vi "write_buffer_to_file.vi"(8 "error in (no error)":errorcluster, 10 "data_logger.lvclass":refnum<class "data_logger.lvclass">, 11 "hydraharp in":refnum<class "hydraharp.lvclass">) -> (0 "error out":errorcluster, 1 "stream_done":bool, 2 "data_logger.lvclass 2":refnum<class "data_logger.lvclass">, 3 "hydraharp out":refnum<class "hydraharp.lvclass">)   [LabVIEW 2015, in "hydraharp.lvclass"]
uses:
  hydraharp.lvclass
  Data Logger Class/data_logger.lvclass
  hydraharp.lvclass/hydraharp.ctl
  lvoop_dll-master/picoquant_Tmodes.ctl
  lvoop_dll-master/picoquant_devices.ctl
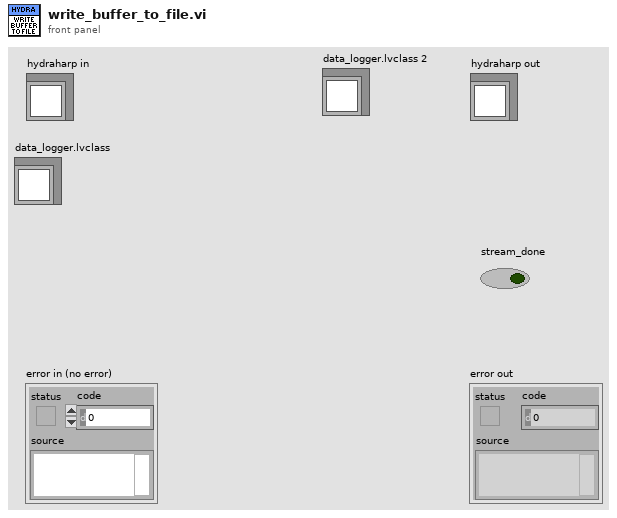
[diagram p1: front panel]
types:
  T1 = typedef "picoquant_devices.ctl" = enum16{"hydraharp", "picoharp"}
  T2 = typedef "hpanel_acq_modes.ctl" = u16
  T3 = typedef "picoquant_Tmodes.ctl" = u16
  T4 = typedef "hydraharp_fifo_queue_data.ctl" = cluster{"fifo_buffer":u32[], "fifo_action":T5}
  T5 = typedef "hydraharp_fifo_actions.ctl" = enum16{"stop", "new_data"}
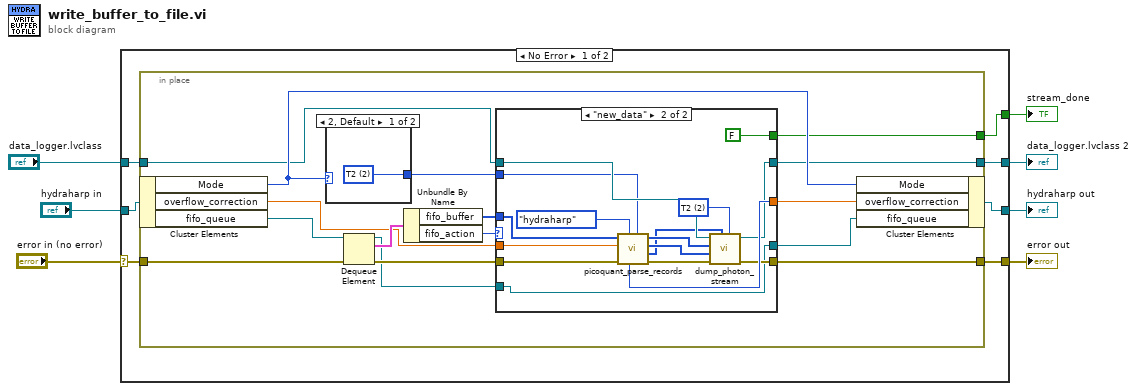
[diagram p0: block diagram]
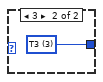
[diagram p2: hidden frame]
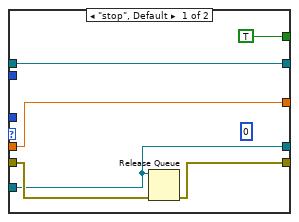
[diagram p3: hidden frame]
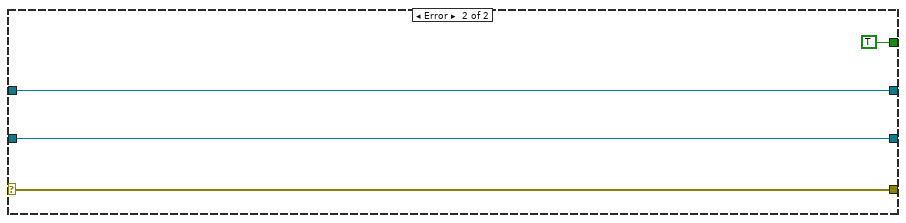
[diagram p4: hidden frame]
diagram:
  n1 = case shown="No Error" "error in (no error)" {
    selector: "error in (no error)" -> [w13 w55]
    tunnel: "data_logger.lvclass" -> [w9 w58]
    tunnel: "hydraharp in" -> [w14 w57]
    tunnel: [w12 w57] -> w4
    tunnel: [w8 w58] -> w3
    tunnel: [w11 TRUE] -> w2
    tunnel: [w10 w55] -> w1
    frame No Error {
      n2 = in-place {
        in-place-border: w13 -> [w29]
        in-place-border: [w20] -> w11
        in-place-border: [w19] -> w10
        in-place-border: w9 -> [w18]
        in-place-border: [w17] -> w8
        n3 = in-place-cluster #1(w14) -> ("Mode"=w21:T2, "overflow_correction"=w25:dbl, "fifo_queue"=w30:refnum<queue>)
        n4 = case shown="2, Default" w21 {
          tunnel: [w31 w32] -> w23
          frame 2, Default {
            w31 = T3 2 items=["T2"=2, "T3"=3] ("acq_mode")
          }
          frame 3 {
            w32 = T3 3 items=["T2"=2, "T3"=3] ("acq_mode")
          }
        }
        n5 = Dequeue Element(queue=w30, error in (no error)=w29) -> (queue out=w16:refnum<queue>, element=w28:T4, error out=w24:errorcluster)  [unwired: 1 in, 1 out]
        n6 = Unbundle By Name(w28) -> ("fifo_buffer"=w26:u32[], "fifo_action"=w27:T5)
        n7 = case shown="\"new_data\"" w27 {
          tunnel: w26 -> [_ w54]
          tunnel: w25 -> [w38 w53]
          tunnel: w24 -> [w35 w52]
          tunnel: w23 -> [_ w41]
          tunnel: [w38 w50] -> w22
          tunnel: [TRUE FALSE] -> w20
          tunnel: [w34 w47] -> w19
          tunnel: w18 -> [w36 w46]
          tunnel: [w36 w45] -> w17
          tunnel: w16 -> [w33 w40]
          tunnel: [w33 w40] -> w15
          frame "stop", Default {
            (unwired) u64 0 ("photon_count")
            n8 = Release Queue(queue=w33, error in (no error)=w35) -> (error out=w34:errorcluster)  [unwired: 1 in, 2 out]
          }
          frame "new_data" {
            w39 = T3 2 items=["T2"=2, "T3"=3] ("acq_mode")
            n9 = call "picoquant_parse_records.vi"("acq_mode"=w41, "Device"=picoquant_devices."hydraharp", "error in (no error)"=w52, "overflow"=w53, "fifo_buffer"=w54) -> ("error out"=w48:errorcluster, "sync"=w42:u64[], "channels"=w43:u8[], "times"=w44:u64[], "overflow"=w50:u64)  [unwired: 1 in, 1 out]
            n10 = call-dynamic "dump_photon_stream.vi"("Ring"=w39, "sync"=w42, "error in (no error)"=w48, "channels"=w43, "photon_records"=w44, "data_logger in"=w46) -> ("error out"=w47:errorcluster, "data_logger out"=w45:refnum<class "data_logger.lvclass">)  [unwired: 4 in]
          }
        }
        n11 = in-place-cluster #1("Mode"=w21, "overflow_correction"=w22, "fifo_queue"=w15) -> (w12:refnum<class "hydraharp.lvclass">)
      }
    }
    frame Error {
    }
  }
  "error out" <- w1
  "hydraharp out" <- w4
  "data_logger.lvclass 2" <- w3
  "stream_done" <- w2
